vi "Pi-Plate VI.vi"(2 "Pi-Plate Command":string, 4 "COM Port":refnum<visa-resource-name>) -> (1 "Bytes Returned":u32, 5 "Output String":string, 7 "Numeric Value":dbl)   [LabVIEW 2025]
uses:
  <vilib>/Instr/_visa.llb/VISA Configure Serial Port (Instr).vi
panel:
  # "Pi-Plates"
  # "Overview: A very simple VI for communicating to Pi-Plates through a serial port.\nRequirements: NI-VISA Driver and a Pi-Plates BRIDGEplate\nInstructions:\n1. Specify the BRIDGEplate COM port in the control below.\n2. Type a single command in the window labeled Pi-Plate Command\n2. Run the VI.\n3. After the command is processed, you will see a reply from the addressed Pi-Plate in the Response window."
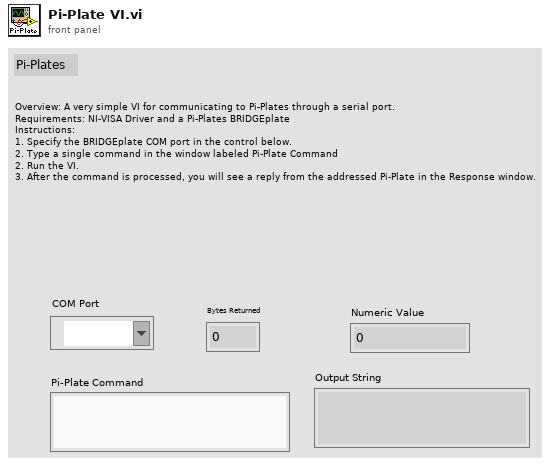
[diagram p1: front panel]
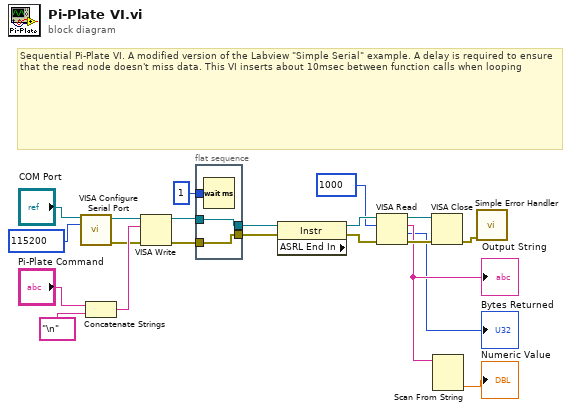
[diagram p0: block diagram]
diagram:
  # "Sequential Pi-Plate VI. A modified version of the Labview \"Simple Serial\" example. A delay is required to ensure that the read node doesn't miss data. This VI inserts about 10msec between function calls when looping"
  n1 = call-poly "VISA Configure Serial Port"("VISA resource name"="COM Port", "baud rate (9600)"=u32 115200) -> ("VISA resource name out"=w13:refnum<visa-resource-name>, "error out"=w12:errorcluster)  [unwired: 7 in, 5 out]
  n2 = Concatenate Strings("Pi-Plate Command", "\n" ("Command")) -> (w19:string)
  n3 = VISA Write(VISA resource name=w13, write buffer=w19, error in (no error)=w12) -> (VISA resource name out=w5:refnum<visa-resource-name>, error out=w3:errorcluster)  [unwired: 1 out]
  n4 = flat-sequence {
    tunnel: w5 -> [w24]
    tunnel: [w24] -> w4
    tunnel: w3 -> [w23]
    tunnel: [w23] -> w2
    tunnel: u32 1 -> [w22]
    frame #0 {
      n5 = Wait (ms)(milliseconds to wait=w22) -> ()  [unwired: 1 out]
    }
  }
  n6 = property class="Instr" props=["ASRL End In"](reference=w4, error in=w2) -> (reference out=w17:refnum<visa-resource-name>, error out=w18:errorcluster)  [unwired: 1 out]
  n7 = VISA Read(VISA resource name=w17, byte count=u32 1000, error in (no error)=w18) -> (VISA resource name out=w15:refnum<visa-resource-name>, read buffer=w8:string, return count=→"Bytes Returned":u32, error out=w14:errorcluster)
  "Output String" <- w8
  n8 = VISA Close(VISA resource name=w15, error in (no error)=w14) -> (error out=w16:errorcluster)
  n9 = Scan From String(input string=w8) -> (output 1=→"Numeric Value":dbl)  [unwired: 4 in, 3 out]
  n10 = call <vilib>:"Simple Error Handler.vi"("error in (no error)"=w16) -> ()  [unwired: 1 in, 8 out]
